vi "Check Valid.vi"(11 "IConfig In":refnum<class "IConfig.lvclass">) -> (3 "Valid?":bool)   [LabVIEW 2019, in "IConfig.lvclass"]
uses:
  IConfig.lvclass
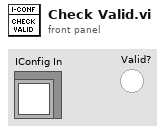
[diagram p1: front panel]
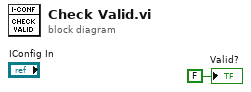
[diagram p0: block diagram]
diagram:
  "Valid?" <- FALSE ("Valid?")
